vi "AlliGator Compute P2 vs P1 Plots.vi"(7 "Lifetime Graph in":refnum<vi>, 8 "error in (no error)":errorcluster, 9 "Phasor Frequency":dbl[unit], 10 "User Selection":T6, 11 "AlliGator IV DVR in":refnum<data-value>) -> (0 "error out":errorcluster, 2 "Message":string, 3 "AlliGator IV DVR out":refnum<data-value>)   [LabVIEW 2021, in "AlliGator Phasor Graph.lvlib"]
doc: "Compute a (P1, P2) scatter plot for all selected phasor plots in the Phasor Graph and send them to the Lifetime & Other Parameters Graph.\n\nP1 & P2 are parameters associated with each plasor plot or derived from the phasor and/or phasor ratio references."
uses:
  AlliGator Phasor Graph.lvlib
  Internal Variables/AlliGator Internal Variables v2.ctl
  <vilib>/vision/Image Controls.llb/IMAQ Image.ctl
  Internal Variables/AlliGator Gate Image Set.ctl
  Files/AlliGator FLI Dataset Type.ctl
  Files/AlliGator Data Series Type.ctl
  Dual-Channel Datasets/AlliGator Dataset Channel.ctl
  Settings/AlliGator Gate Arithmetic.ctl
  Source Image/AlliGator Displayed Image.ctl
  Image/Named ROI Description.ctl
  AlliGator Decay Metadata v3.ctl
  Decay Analysis/Decay Preprocessing/AlliGator Decay Background Subtraction Info.ctl
  Decay Analysis/Decay Preprocessing/AlliGator Baseline Subtraction Method.ctl
  Graphs/XY Graph/XY Graph Plot Shift Parameters.ctl
  Graphs/XY Graph/XY Graph Plot Shift Method.ctl
  Decay Analysis/Decay Preprocessing/AlliGator Decay Extrapolation Parameters.ctl
  Phasor/Calibration Phasor (m, phi).ctl
  Phasor/Phasor Reference Series.ctl
  Phasor/Phasor Calibration Map v2.ctl
  Phasor/Phasor (g, s).ctl
  AlliGator Raw Phasor Plot Data v4.ctl
  Phasor/Phasor Standard Deviation Options.ctl
  Phasor Plot/AlliGator Phasor Multi-Harmonic Data.ctl
  Phasor/Phasor Harmonic Data.ctl
  Decay Fit Parameter Map/AlliGator Decay Fit Options & Parameters v2.ctl
  Fits/IRF(X)PSED/Decay Fit Options v2.ctl
  Fits/Decay Convolution/Decay Model.ctl
  Fits/Residual Type.ctl
  Fits/IRF(X)PSED/Fit Weights Type.ctl
  Fits/Non-linear Fitting Method v2.ctl
  Fits/Fit Calculation Method.ctl
  Fits/Non-linear Fitting Algorithm.ctl
  Decay Analysis/Decay Fit/AlliGator Decay Fit Parameter Constraints 2.ctl
  Fits/IRF(X)PSED/Decay Fit Parameters In List.ctl
  Fits/IRF(X)PSED/MLE Baseline Offset Type.ctl
  Decay Analysis/Decay Preprocessing/AlliGator Decay Preprocessing Parameters.ctl
  Fits/IRF(X)PSED/Decay Fit Parameters & Derived Quantities List v2.ctl
  Decay Fit Parameter Map/AlliGator Parameter Maps Data.ctl
  Graphs/XY Graph/XY Graph Selected Plot Info.ctl
  Graphs/XY Graph/XY Graph Refnum.ctl
  <vilib>/Utility/miscctls.llb/LVPoint32TypeDef.ctl
  AlliGator Phasor Plot Scatter Plot Parameters.ctl
  AlliGator Phasor Graph Parameter List.ctl
  <userlib>/_OpenG.lib/array/array.llb/Filter 1D Array with Scalar (I32)__ogtk.vi
  Graphs/XY Graph/XY Graph Add Single Plot with Name.vi
  Graphs/XY Graph/XY Graph Add-Ons.lvlib
  Strings/Strings.lvlib
  <userlib>/_OpenG.lib/array/array.llb/openg_array.lvlib
  Phasor/Phasor.lvlib
  Image/Image.lvlib
  Decay Analysis/Decay Preprocessing/AlliGator Decay Preprocessing.lvlib
  Files/AlliGator Files.lvlib
  Internal Variables/AlliGator Internal Variables.lvlib
  Phasor Plot/AlliGator Phasor Plot.lvlib
  Source Image/AlliGator Source Image.lvlib
  Fits/Fits.lvlib
  Decay Analysis/Decay Fit/AlliGator Decay Fit.lvlib
  Decay Fit Parameter Map/AlliGator Decay Fit Parameter Map.lvlib
  Settings/AlliGator Settings.lvlib
  Dual-Channel Datasets/AlliGator Dual-Channel Datasets.lvlib
panel:
  # "vs"
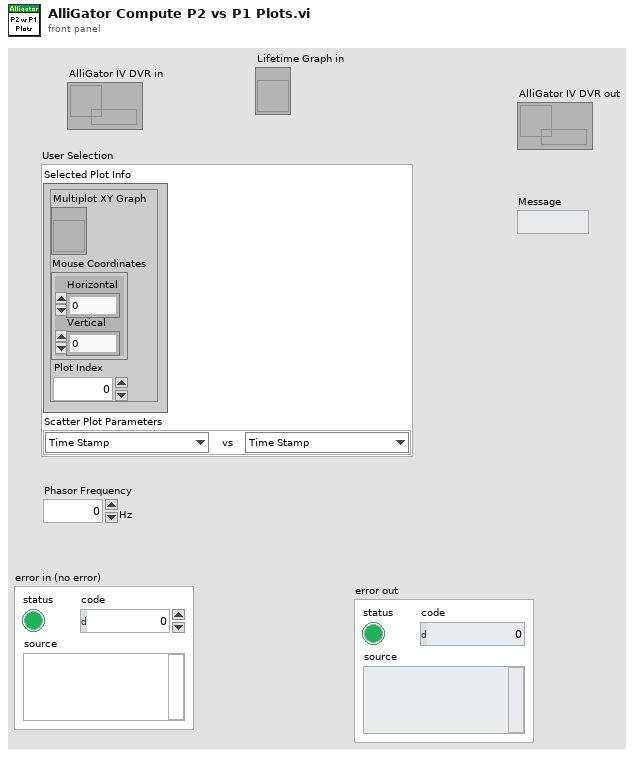
[diagram p1: front panel]
types:
  T1 = typedef "XY Graph Add-Ons.lvlib/XY Graph Selected Plot Info.ctl" = cluster{"Multiplot XY Graph":T2, "Mouse Coordinates":T3, "Plot Index":i32}
  T2 = typedef "XY Graph Add-Ons.lvlib/XY Graph Refnum.ctl" = refnum<vi>
  T3 = typedef "LVPoint32TypeDef.ctl" = cluster{"Horizontal":i32, "Vertical":i32}
  T4 = typedef "AlliGator Phasor Graph.lvlib/AlliGator Phasor Plot Scatter Plot Parameters.ctl" = cluster{"Parameter 2":T5, "Parameter 1":T5}
  T5 = typedef "AlliGator Phasor Graph.lvlib/AlliGator Phasor Graph Parameter List.ctl" = enum16{"Time Stamp", "Index", "Phasor Parameters", "Phasor g", "Phasor s", "Phasor phi", "Phasor m", "Modulus Lifetime", "Phase Lifetime", "ROI Parameters", "ROI Center x", "ROI Center y", "ROI # pixels ", "Decay Parameters", "Intensity", "Background/Gate", "Intensity - Background", "Fitted Lifetime", "Fitted Intensity", "Phasor Ratio Parameters", "Amplitude Phasor Ratio", "Intensity Phasor Ratio", "Amplitude-Averaged Lifetime", "Intensity-Averaged Lifetime", "-", "Phasor Parameters SDV", "Phasor g SDV", "Phasor s SDV", "Phasor phi SDV", "Phasor m SDV", "Phase Lifetime SDV", "Modulus Lifetime SDV", "Phasor Ratio Parameters SDV", "Amplitude Phasor Ratio SDV", "Intensity Phasor Ratio SDV", "Amplitude-Averaged Lifetime SDV", "Intensity-Averaged Lifetime SDV"}
  T6 = cluster{"Selected Plot Info":T1, "Scatter Plot Parameters":T4}
  T7 = typedef "XY Graph Add-Ons.lvlib/XY Plot Data.ctl" = cluster{"X Array":dbl[], "Y Array":dbl[]}
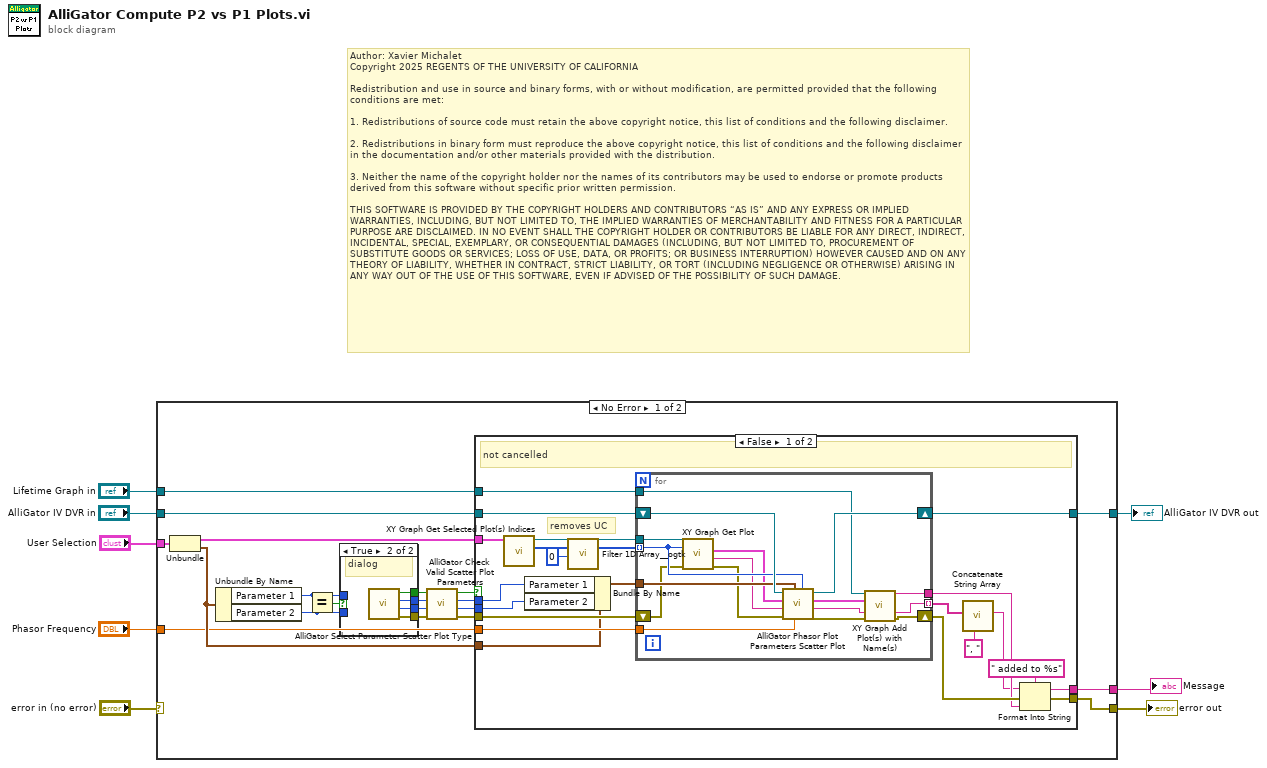
[diagram p0: block diagram]
diagram:
  # "Author: Xavier Michalet\nCopyright 2025 REGENTS OF THE UNIVERSITY OF CALIFORNIA\n\nRedistribution and use in source and binary forms, with or without modification, are permitted provided that the following conditions are met:\n\n1. Redistributions of source code must retain the above copyright notice, this list of conditions and the following disclaimer.\n\n2. Redistributions in binary form must reproduce the above copyright notice, this list of conditions and the following disclaimer in the documentation and/or other materials provided with the distribution.\n\n3. Neither the name of the copyright holder nor the names of its contributors may be used to endorse or promote products derived from this software without specific prior written permission.\n\nTHIS SOFTWARE IS PROVIDED BY THE COPYRIGHT HOLDERS AND CONTRIBUTORS “AS IS” AND ANY EXPRESS OR IMPLIED WARRANTIES, INCLUDING, BUT NOT LIMITED TO, THE IMPLIED WARRANTIES OF MERCHANTABILITY AND FITNESS FOR A PARTICULAR PURPOSE ARE DISCLAIMED. IN NO EVENT SHALL THE COPYRIGHT HOLDER OR CONTRIBUTORS BE LIABLE FOR ANY DIRECT, INDIRECT, INCIDENTAL, SPECIAL, EXEMPLARY, OR CONSEQUENTIAL DAMAGES (INCLUDING, BUT NOT LIMITED TO, PROCUREMENT OF SUBSTITUTE GOODS OR SERVICES; LOSS OF USE, DATA, OR PROFITS; OR BUSINESS INTERRUPTION) HOWEVER CAUSED AND ON ANY THEORY OF LIABILITY, WHETHER IN CONTRACT, STRICT LIABILITY, OR TORT (INCLUDING NEGLIGENCE OR OTHERWISE) ARISING IN ANY WAY OUT OF THE USE OF THIS SOFTWARE, EVEN IF ADVISED OF THE POSSIBILITY OF SUCH DAMAGE."
  n1 = case shown="No Error" "error in (no error)" {
    selector: "error in (no error)" -> [_ w77]
    tunnel: [w21 w77] -> w8
    tunnel: "Lifetime Graph in" -> [w20 _]
    tunnel: "Phasor Frequency" -> [w19 _]
    tunnel: [w17 _] -> w5
    tunnel: [w14 w76] -> w4
    tunnel: "AlliGator IV DVR in" -> [w13 w76]
    tunnel: "User Selection" -> [w11 _]
    frame No Error {
      n2 = Unbundle(w11) -> ("Selected Plot Info"=w9:T1, "Scatter Plot Parameters"=w28:T4)
      n3 = Unbundle By Name(w28) -> ("Parameter 1"=w23:T5, "Parameter 2"=w24:T5)
      n4 = Equal?(x=w23, y=w24) -> (x = y?=w22:bool)
      n5 = case shown="True" w22 {
        tunnel: [_ w34] -> w12
        tunnel: [w30 w33] -> w15
        tunnel: [w29 w32] -> w16
        tunnel: [_ w31] -> w18
        tunnel: w23 -> [w30 _]
        tunnel: w24 -> [w29 _]
        frame False {
          # "programmatic"
        }
        frame True {
          # "dialog"
          n6 = call "AlliGator Select Parameter Scatter Plot Type.vi"() -> ("Error Out"=w34:errorcluster, "Parameter 2"=w32:T5, "Parameter 1"=w33:T5, "Cancelled?"=w31:bool)  [unwired: 8 in]
        }
      }
      n7 = call "AlliGator Check Valid Scatter Plot Parameters.vi"("error in (no error)"=w12, "Parameter 2"=w16, "Parameter 1"=w15, "Cancelled?"=w18) -> ("error out"=w10:errorcluster, "Parameter 2"=w26:T5, "Parameter 1"=w25:T5, "Cancelled?"=w27:bool)  [unwired: 4 in]
      n8 = case shown="False" w27 {
        tunnel: w10 -> [w56 w74]
        tunnel: w13 -> [w55 w75]
        tunnel: [w54 w75] -> w14
        tunnel: w25 -> [w53 _]
        tunnel: w26 -> [w52 _]
        tunnel: [w48 _] -> w17
        tunnel: w19 -> [w50 _]
        tunnel: w20 -> [w49 _]
        tunnel: [w46 w74] -> w21
        tunnel: w28 -> [w42 _]
        tunnel: w9 -> [w41 _]
        frame False {
          # "removes UC"
          # "not cancelled"
          n9 = call "XY Graph Get Selected Plot(s) Indices.vi"("Selected Plot Info"=w41) -> ("Plot(s) at Coordinates"=w37:i32[], "XYGraph out"=w38:T2)  [unwired: 7 in, 2 out]
          n10 = Bundle By Name(cluster=w42, "Parameter 1"=w53, "Parameter 2"=w52) -> (w51:T4)
          n11 = call-poly <userlib>:"Filter 1D Array__ogtk.vi"("items to filter"=0, "array"=w37) -> ("filtered array"=w35:i32[])  [unwired: 4 in, 1 out]
          n12 = for {
            tunnel: w51 -> [w71]
            tunnel: w50 -> [w70]
            tunnel: w49 -> [w68]
            tunnel: [w65] -> w45 mode=indexing
            shift-right: [w66] -> w47
            shift-left: w56 -> [w60]
            shift-right: [w72] -> w54
            shift-left: w55 -> [w73]
            tunnel: [w64] -> w43
            tunnel: w38 -> [w62]
            tunnel: w35 -> [w61] mode=indexing
            n13 = call "XY Graph Get Plot.vi"("error in (no error)"=w60, "Plot Index (-1: last)"=w61, "XYGraph in"=w62) -> ("error out"=w59:errorcluster, "Plot Name"=w57:string, "Plot Data"=w58:T7)  [unwired: 4 in, 2 out]
            n14 = call "AlliGator Phasor Plot Parameters Scatter Plot.vi"("Phasor Plot Idx"=w61, "Phasor Frequency"=w70, "Scatter Plot Parameters"=w71, "error in (no error)"=w59, "PhasorPlot Name in"=w57, "Phasor Plot Data"=w58, "AlliGator IV DVR in"=w73) -> ("error out"=w69:errorcluster, "Plot Name out"=w67:string, "Parameters Scatter Plot"=w63:T7, "AlliGator IV DVR out"=w72:refnum<data-value>)  [unwired: 1 in]
            n15 = call-poly "XY Graph Add Plot(s) with Name(s).vi"("XYGraph Ref in"=w68, "Plot"=w63, "Plot Name (\"Plot\")"=w67, "error in (no error)"=w69) -> ("XY Graph Caption (or Label)"=w64:string, "Plot Name"=w65:string, "error out"=w66:errorcluster)  [unwired: 8 in, 1 out]
          }
          n16 = call "Concatenate String Array.vi"("Separator (TAB)"=", ", "String Array"=w45) -> ("Formatted String"=w40:string)  [unwired: 9 in]
          n17 = Format Into String(format string=" added to %s", initial string=w40, error in=w47, w43) -> (resulting string=w48:string, error out=w46:errorcluster)
        }
        frame True {
          # "Cancelled"
        }
      }
    }
    frame Error {
    }
  }
  "error out" <- w8
  "Message" <- w5
  "AlliGator IV DVR out" <- w4
